vi "tcptest.vi"() -> ()   [LabVIEW 2019]
panel:
  out "Waveform Chart 3":waveform(dbl)(graph)
  out "output array":dbl[](array[numeric])
  out "Waveform Chart 2":waveform(dbl)(graph)
  out "Waveform Chart":waveform(dbl)(graph)
  out "current time":timestamp
  in  "stop":bool
  out "Slave Input Registers 2":i32[](array[numeric]) caption="Slave Input Registers (Read Only)"
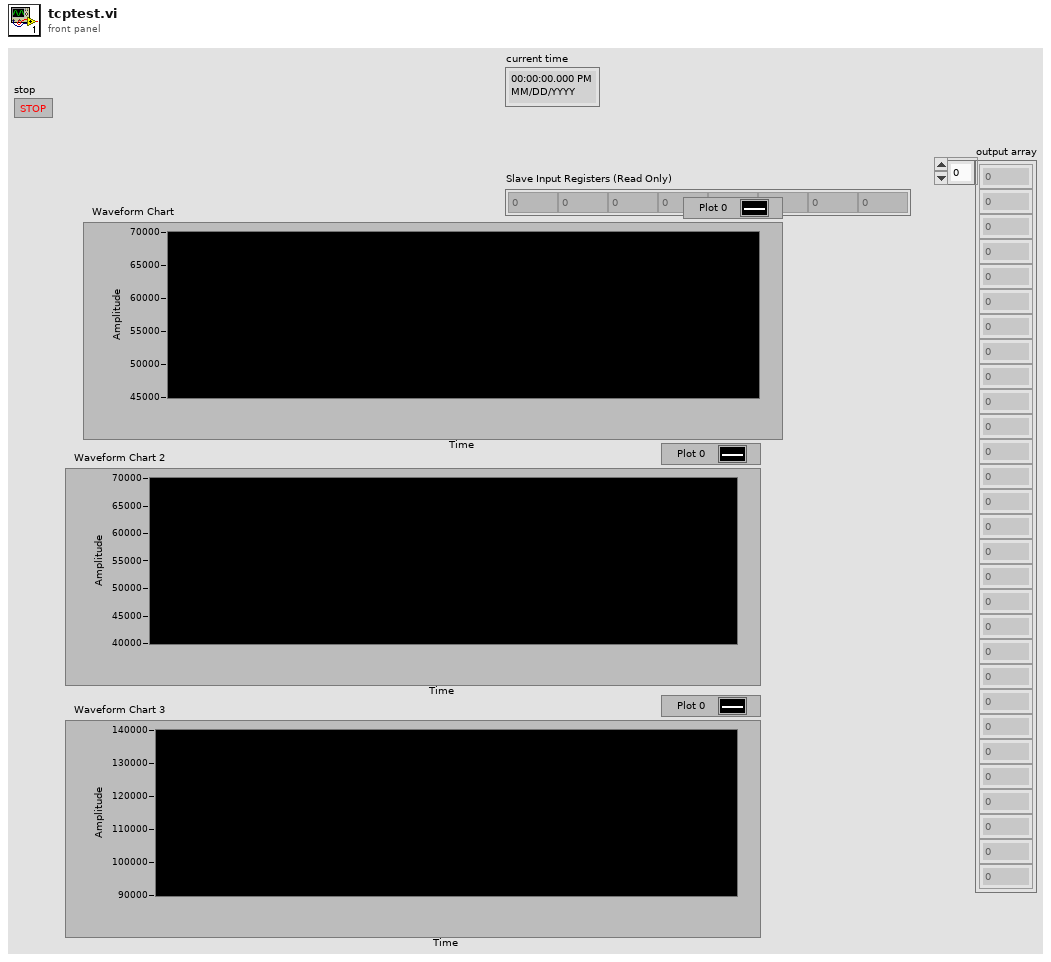
[diagram p1: front panel]
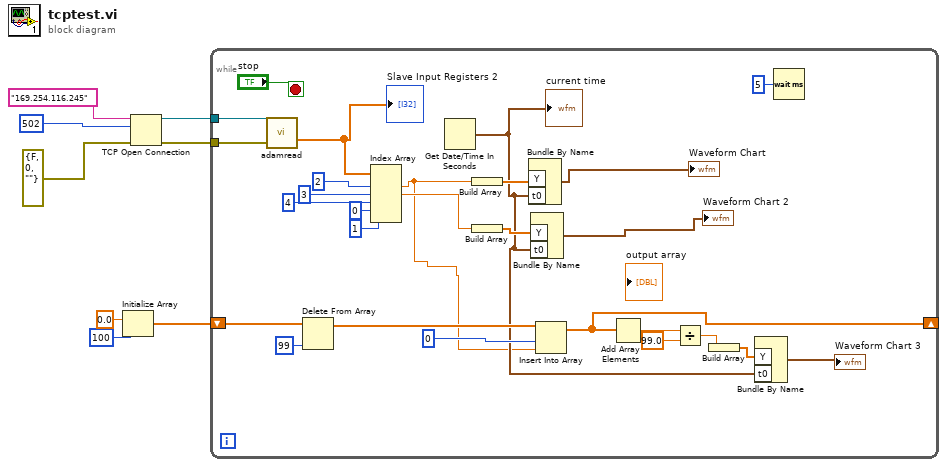
[diagram p0: block diagram]
diagram:
  n1 = Initialize Array(0.0 ("element"), 100 ("dimension size")) -> (w1:dbl[])
  n2 = TCP Open Connection(address="169.254.116.245", remote port or service name=u16 502, error in (no error)=errorcluster {"status"=FALSE, "code"=0, "source"=""}) -> (connection ID=w6:refnum<k5>, error out=w5:errorcluster)  [unwired: 2 in]
  n3 = while {
    tunnel: w6 -> [w35]
    tunnel: w5 -> [w34]
    shift-right: [w15] -> _
    shift-left: w1 -> [w21]
    stop <- "stop" stop-if-true
    n4 = call "adamread.vi"("TCP Connection Refnum in"=w35, "error in (no error)"=w34) -> ("Slave Input Registers 2"=w32:dbl[])  [unwired: 11 in, 2 out]
    "Slave Input Registers 2" <- w32
    n5 = Delete From Array(array=w21, index=99) -> (array with subset deleted=w19:dbl[])  [unwired: 1 in, 1 out]
    n6 = Index Array(array=w32, index #1=2 ("index"), index #2=3 ("index"), index #3=4 ("index"), index #4=0 ("index"), index #5=1 ("index")) -> (element #1=w9:dbl, element #2=w10:dbl)  [unwired: 3 out]
    n7 = Get Date/Time In Seconds() -> (seconds since 1Jan1904=w12:timestamp)
    "current time" <- w12
    n8 = Build Array(w9) -> (w26:dbl[])
    n9 = Build Array(w10) -> (w24:dbl[])
    n10 = Bundle By Name("Y"=w26, "t0"=w12) -> (→"Waveform Chart":waveform(dbl))  [unwired: 1 in]
    n11 = Bundle By Name("Y"=w24, "t0"=w12) -> (→"Waveform Chart 2":waveform(dbl))  [unwired: 1 in]
    n12 = Insert Into Array(array=w19, index=0, new element=w9) -> (w15:dbl[])
    n13 = Add Array Elements(numeric array=w15) -> (sum=w17:dbl)
    n14 = Divide(x=w17, y=99.0) -> (x/y=w14:dbl)
    n15 = Build Array(w14) -> (w13:dbl[])
    n16 = Bundle By Name("Y"=w13, "t0"=w12) -> (→"Waveform Chart 3":waveform(dbl))  [unwired: 1 in]
    n17 = Wait (ms)(milliseconds to wait=u32 5) -> ()  [unwired: 1 out]
  }
